vi "Software Update HCC Display Missing Newfis in String Format.vi"(11 "Newfi Array":string[][](array[string])) -> (3 "Newfi Concatenated String":string)   [LabVIEW 2014]
panel:
  out "size(s)":i32
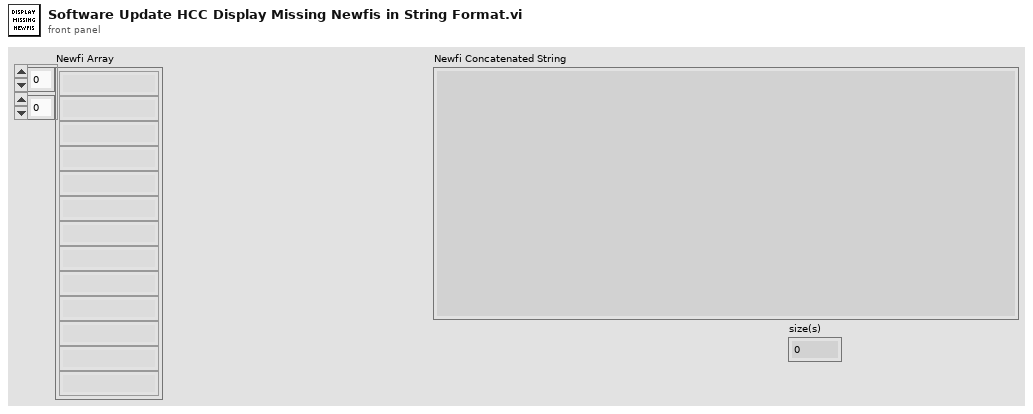
[diagram p1: front panel]
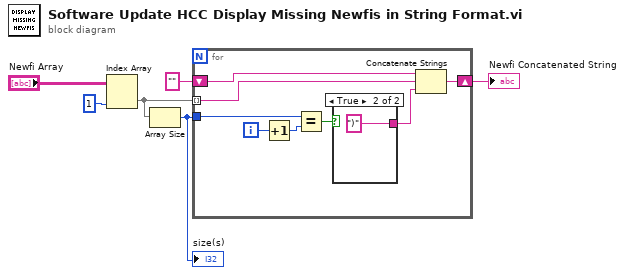
[diagram p0: block diagram]
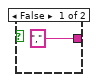
[diagram p2: hidden frame]
diagram:
  n1 = Index Array(array="Newfi Array", index (col)=1 ("disabled index (col)")) -> (element=w2:string[])  [unwired: 1 in]
  n2 = Array Size(array=w2) -> (size(s)=w1:i32)
  "size(s)" <- w1
  n3 = for {
    tunnel: w2 -> [w13] mode=indexing
    shift-right: [w11] -> w6
    shift-left: "" -> [w14]
    tunnel: w1 -> [w9]
    i -> [w10]
    n4 = Increment(x=w10) -> (x+1=w8:i32)
    n5 = Equal?(x=w9, y=w8) -> (x = y?=w7:bool)
    n6 = case shown="True" w7 {
      tunnel: ["," ("string") ")" ("string")] -> w12
      frame False {
      }
      frame True {
      }
    }
    n7 = Concatenate Strings(w14, w13, w12) -> (w11:string)
  }
  "Newfi Concatenated String" <- w6
